vi "Display Results.vi"(8 "error in (no error)":errorcluster, 10 "Results.lvclass":refnum<class "Results.lvclass">, 11 "Operator UI in":refnum<class "Controller UI.lvclass">) -> (0 "error out":errorcluster, 3 "Operator UI out":refnum<class "Controller UI.lvclass">)   [LabVIEW 2016, in "Controller UI.lvlib" / "Controller UI.lvclass"]
uses:
  <userlib>/Common Components/Controller UI/Controller UI.lvclass
  C:/Program Files (x86)/National Instruments/LabVIEW 2016/user.lib/Common Components/User Interface/UI.lvclass
  <userlib>/Common Components/Results/Results.lvclass
  <userlib>/Common Components/Controller UI/Controller UI.lvclass/Controller UI.ctl
  <userlib>/Common Components/Results/Results.lvclass/Results.ctl
  <userlib>/Common Components/Controller UI/Accessors/Read Results Listbox.vi
  <userlib>/Common Components/User Interface/UI.lvclass
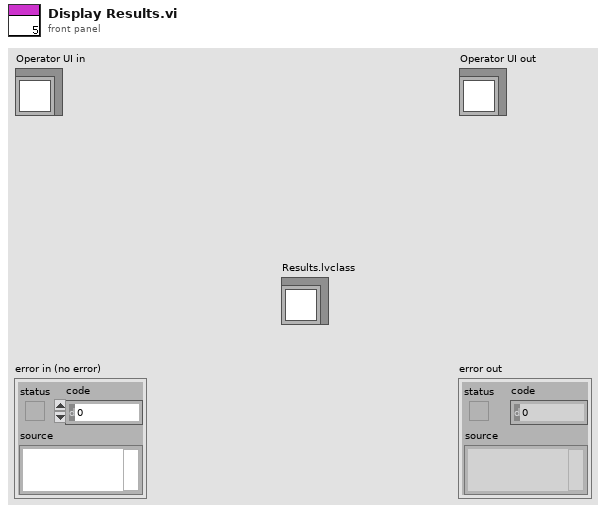
[diagram p1: front panel]
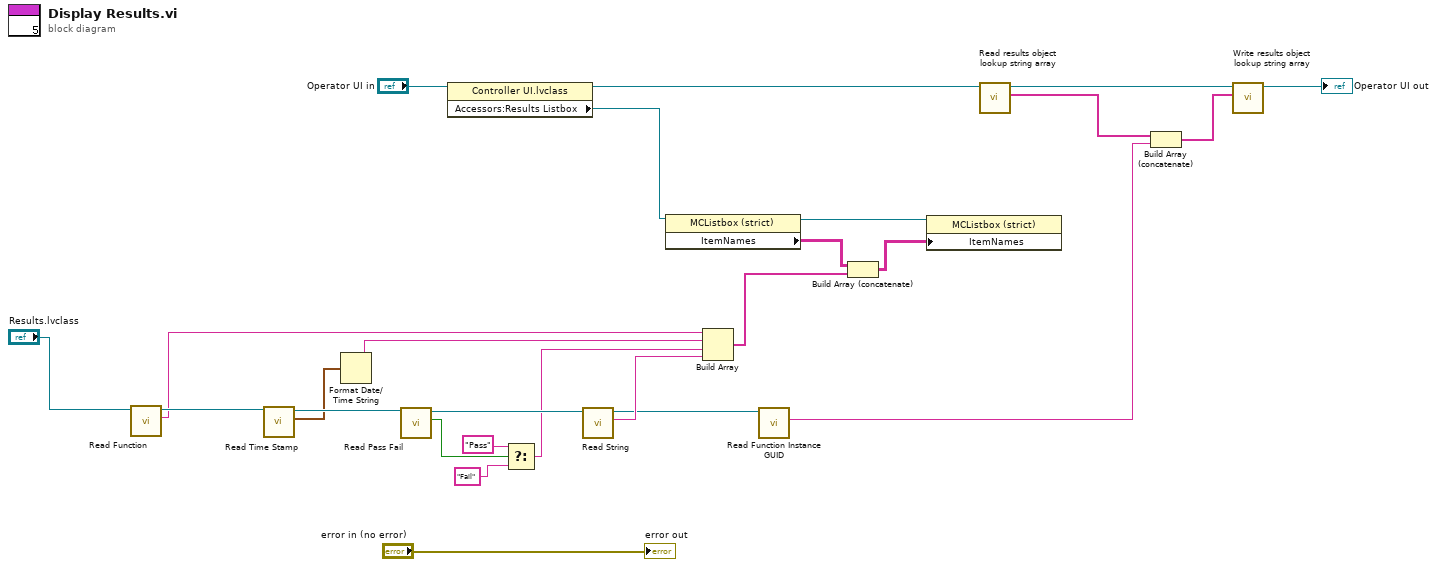
[diagram p0: block diagram]
diagram:
  n1 = call <userlib>:"Read Function.vi"("Results in"="Results.lvclass") -> ("Function"=w12:string, "Results out"=w13:refnum<class "Results.lvclass">)  [unwired: 8 in, 1 out]
  n2 = call <userlib>:"Read Time Stamp.vi"("Results in"=w13) -> ("Time Stamp"=w9:timestamp, "Results out"=w14:refnum<class "Results.lvclass">)  [unwired: 8 in, 1 out]
  n3 = Format Date/Time String(seconds (now)=w9) -> (date/time string=w10:string)  [unwired: 2 in]
  n4 = call <userlib>:"Read Pass Fail.vi"("Results in"=w14) -> ("Pass Fail"=w18:bool, "Results out"=w19:refnum<class "Results.lvclass">)  [unwired: 8 in, 1 out]
  n5 = property class="Controller UI.lvclass"(reference="Operator UI in") -> (reference out=w2:refnum<class "Controller UI.lvclass">, "Accessors:Results Listbox"=w1:refnum<vi>)  [unwired: 1 in, 1 out]
  n6 = Select(t="Pass" ("element"), s=w18, f="Fail" ("element")) -> (s? t:f=w15:string)
  n7 = call <userlib>:"Read String.vi"("Results in"=w19) -> ("String"=w20:string, "Results out"=w4:refnum<class "Results.lvclass">)  [unwired: 8 in, 1 out]
  n8 = property class="MCListbox (strict)"(reference=w1) -> (reference out=w24:refnum<vi>, "ItemNames"=w23:string[][])  [unwired: 1 in, 1 out]
  n9 = Build Array(w12, w10, w15, w20) -> (w21:string[])
  n10 = call <userlib>:"Read Function Instance GUID.vi"("Results in"=w4) -> ("Function Instance GUID"=w3:string)  [unwired: 8 in, 2 out]
  n11 = Build Array (concatenate)(w23, w21) -> (w22:string[][])
  n12 = property class="MCListbox (strict)"(reference=w24, "ItemNames"=w22) -> ()  [unwired: 1 in, 2 out]
  n13 = call <userlib>:"Read results object lookup string array.vi"("UI in"=w2) -> ("results object lookup string array"=w6:string[], "UI out"=w8:refnum<class "Controller UI.lvclass">)  [unwired: 8 in, 1 out]
  n14 = Build Array (concatenate)(w6, w3) -> (w5:string[])
  n15 = call <userlib>:"Write results object lookup string array.vi"("results object lookup string array"=w5, "UI in"=w8) -> ("UI out"=→"Operator UI out":refnum<class "Controller UI.lvclass">)  [unwired: 8 in, 1 out]
  "error out" <- "error in (no error)"
